vi "Get System Info - Example.vi"() -> ()   [LabVIEW 2015, in "SMI.lvlib"]
uses:
  SMI.lvlib
  classes/Controller/Controls/ControllerInformation.ctl
  classes/Controller/Controls/DeviceInformation.ctl
  classes/Controller/Controls/NetworkAdapterSettings.ctl
  classes/Chassis/Controls/ChassisInformation.ctl
  classes/Module/Controls/ModuleInformation.ctl
  classes/SysCfg Device/SysCfg Device.lvclass
  classes/Controller/Controller.lvclass
  classes/Chassis/Chassis.lvclass
  classes/Device/Device.lvclass
  classes/Module/Module.lvclass
panel:
  out "Chassis Information":T3 {"Remote Chassis"."Modules"."Module Code" format="%.0x"; "Local Chassis"."Modules"."Module Code" format="%.0x"; "Local Chassis"."Chassis"."Product ID" format="%.0x"}
  out "error out":errorcluster
  out "Controller Information":T4={"System Hardware Reference"=refnum, "Vendor Name"="", "Product Name"="", "Product ID"=0, "Serial Number"="", "Device Information"={"Resource"="", "Device Class"="", "System Start Time"=timestamp(0 s since 1904-01-01), "Current Time"=timestamp(0 s since 1904-01-01), "Time Zone"="", "Firmware Revision"="", "Image Title"="", "Image Version"="", "System Status"=""}, "Primary Network Adapter"={"IP Address"="", "MAC Address"="", "IP Address Request Mode"=1, "SubnetMask"="", "Gateway"="", "DNS Server"="", "Adapter Mode"=1, "Adapter Type"=1}, "Secondary Network Adapters"=[]} {"Product ID" format="%.0x"; "Primary Network Adapter"."IP Address Request Mode" items=["Static"=1, "DHCP/Link Local"=2, "Link-Local Only"=4, "DHCP Only"=8]; "Primary Network Adapter"."Adapter Type" items=["Ethernet"=1, "WLAN"=2]; "Primary Network Adapter"."Adapter Mode" items=["Disabled"=1, "TCP/IP Ethernet"=2, "Deterministic"=4, "EtherCAT"=8, "TCP/IP WLAN Connect"=32, "TCP/IP WLAN Create"=64]; "Secondary Network Adapters"."IP Address Request Mode" items=["Static"=1, "DHCP/Link Local"=2, "Link-Local Only"=4, "DHCP Only"=8]; "Secondary Network Adapters"."Adapter Type" items=["Disabled"=1, "TCP/IP Ethernet"=2, "Deterministic"=4, "EtherCAT"=8, "TCP/IP WLAN Connect"=32, "TCP/IP WLAN Create"=64]; "Secondary Network Adapters"."Adapter Mode" items=["Disabled"=1, "TCP/IP Ethernet"=2, "Deterministic"=4, "EtherCAT"=8, "TCP/IP WLAN Connect"=32, "TCP/IP WLAN Create"=64]}
  in  "NI Auth":cluster{"User Name":string, "Password":string}[](array[cluster])
  in  "Target Address":string
  # "NI Auth default settings \n(username: admin, \npassword: <blank>) are\nattempted automatically."
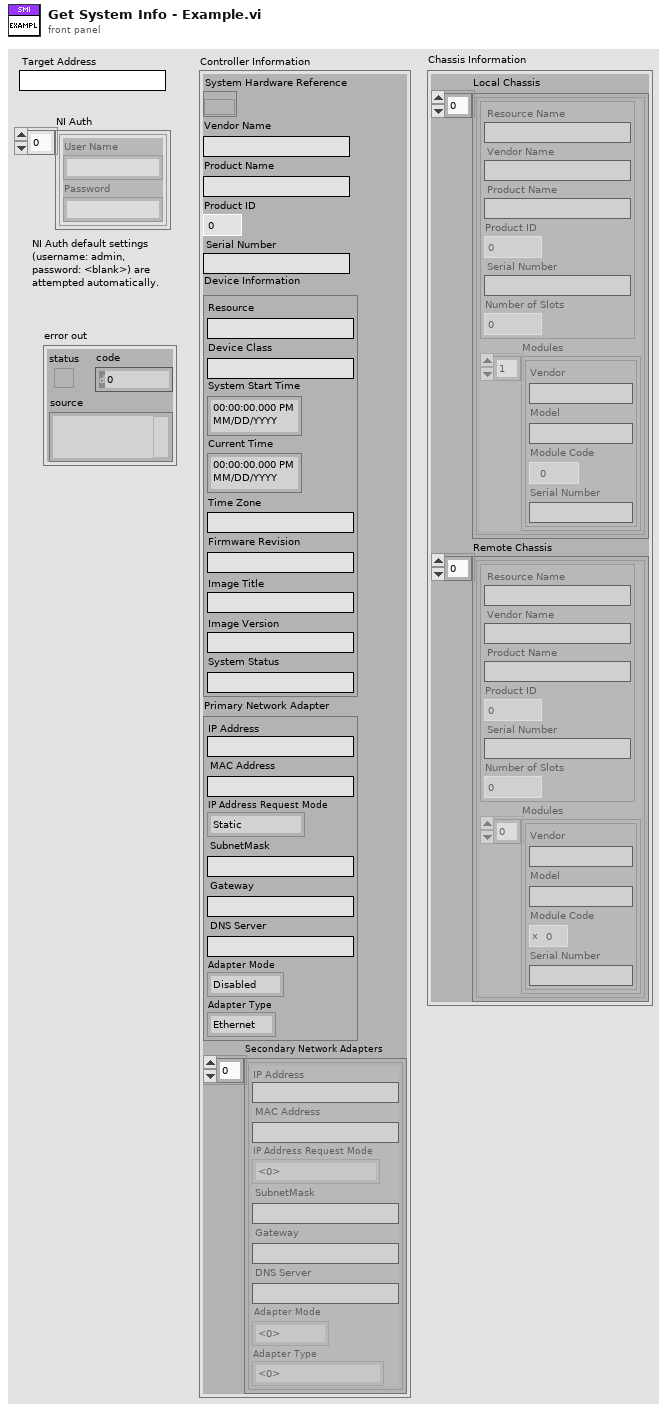
[diagram p1: front panel]
types:
  T1 = typedef "SMI.lvlib/Chassis.lvclass/ChassisInformation.ctl" = cluster{"Resource Name":string, "Vendor Name":string, "Product Name":string, "Product ID":u32, "Serial Number":string, "Number of Slots":i32}
  T2 = typedef "SMI.lvlib/Module.lvclass/ModuleInformation.ctl" = cluster{"Vendor":string, "Model":string, "Module Code":u16, "Serial Number":string}
  T3 = cluster{"Local Chassis":cluster{"Chassis":T1, "Modules":T2[]}[], "Remote Chassis":cluster{"Chassis":T1, "Modules":T2[]}[]}
  T4 = typedef "SMI.lvlib/Controller.lvclass/ControllerInformation.ctl" = cluster{"System Hardware Reference":refnum<k20>, "Vendor Name":string, "Product Name":string, "Product ID":u16, "Serial Number":string, "Device Information":T5, "Primary Network Adapter":T6, "Secondary Network Adapters":T6[]}
  T5 = typedef "SMI.lvlib/Controller.lvclass/DeviceInformation.ctl" = cluster{"Resource":string, "Device Class":string, "System Start Time":timestamp, "Current Time":timestamp, "Time Zone":string, "Firmware Revision":string, "Image Title":string, "Image Version":string, "System Status":string}
  T6 = typedef "SMI.lvlib/Controller.lvclass/NetworkAdapterSettings.ctl" = cluster{"IP Address":string, "MAC Address":string, "IP Address Request Mode":u32, "SubnetMask":string, "Gateway":string, "DNS Server":string, "Adapter Mode":u32, "Adapter Type":u32}
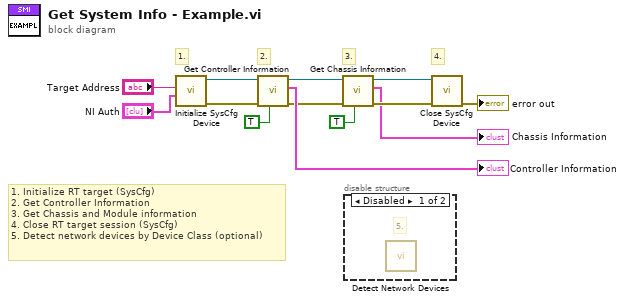
[diagram p0: block diagram]
diagram:
  # "4."
  # "3."
  # "2."
  # "1."
  # "1. Initialize RT target (SysCfg)\n2. Get Controller Information\n3. Get Chassis and Module information\n4. Close RT target session (SysCfg)\n5. Detect network devices by Device Class (optional)"
  n1 = call "Initialize SysCfg Device.vi"("NI Auth"="NI Auth", "Target Address"="Target Address") -> ("error out"=w5:errorcluster, "Controller out"=w6:refnum<class "Controller.lvclass">)  [unwired: 8 in]
  n2 = call "Get Controller Information.vi"("Network Adapters (F)"=TRUE ("Network Adapters"), "error in"=w5, "Controller in"=w6) -> ("error out"=w2:errorcluster, "Device Information"=→"Controller Information":T4, "Controller out"=w3:refnum<class "Controller.lvclass">)  [unwired: 6 in]
  n3 = call "Get Chassis Information.vi"("Detect Modules (F)"=TRUE, "error in"=w2, "Controller in"=w3) -> ("error out"=w10:errorcluster, "Chassis Information"=→"Chassis Information":T3, "Controller out"=w9:refnum<class "Controller.lvclass">)  [unwired: 6 in]
  n4 = disable-structure shown="Disabled" {
    frame Disabled {
      # "5."
      n5 = call "Detect Network Devices.vi"() -> ()  [unwired: 8 in, 4 out]
    }
    frame Enabled {
    }
  }
  n6 = call "Close SysCfg Device.vi"("error in"=w10, "Controller in"=w9) -> ("error out"=→"error out":errorcluster)  [unwired: 9 in]
